vi "Write maxFailTPDOCounter.vi"(8 "error in (no error)":errorcluster, 10 "maxFailTPDOCounter":u8, 11 "OrionBMSClass in":refnum<class "OrionBMSClass.lvclass">) -> (0 "error out":errorcluster, 3 "OrionBMSClass out":refnum<class "OrionBMSClass.lvclass">)   [LabVIEW 2018, in "OrionBMSClass.lvclass"]
uses:
  OrionBMSClass.lvclass
  OrionBMSClass.lvclass/OrionBMSClass.ctl
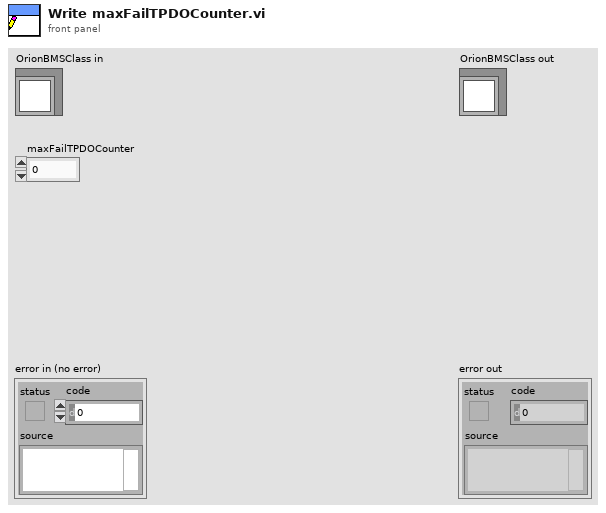
[diagram p1: front panel]
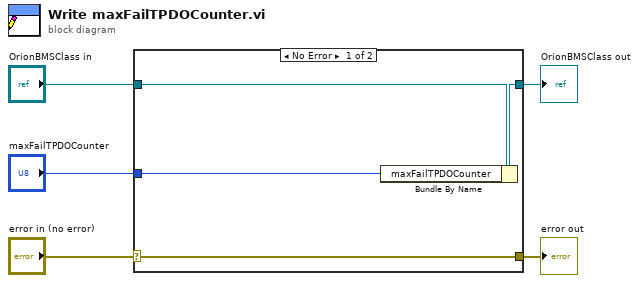
[diagram p0: block diagram]
diagram:
  n1 = case shown="No Error" "error in (no error)" {
    selector: "error in (no error)" -> [w9 w10]
    tunnel: [w9 w10] -> w4
    tunnel: [w7 w11] -> w2
    tunnel: "OrionBMSClass in" -> [w8 w11]
    tunnel: "maxFailTPDOCounter" -> [w6 _]
    frame No Error {
      n2 = Bundle By Name(cluster=w8, "maxFailTPDOCounter"=w6) -> (w7:refnum<class "OrionBMSClass.lvclass">)
    }
    frame Error {
    }
  }
  "error out" <- w4
  "OrionBMSClass out" <- w2
